vi "CC_FPGA_main.vi"() -> ()   [LabVIEW 2019]
uses:
  <vilib>/FPGAPlugInAG/sbRIO-9627/niLvFpga_Open_sbRIO-9627.vi
  <vilib>/rvi/interface/common/dynamic/niFpgaDynamicAddResources.vi
  <vilib>/Utility/error.llb/Error Cluster From Error Code.vi
  <vilib>/rvi/errors/niLvFpgaAdjustHostInterfaceError.vi
  <vilib>/FPGAPlugInAG/Dynamic/niLvFpga_Close_Dynamic.vi
  <vilib>/rvi/interface/nirviOpenFPGA/nirviOpenFPGA.xnode
  FPGA Bitfiles/ccmultiplier_FPGATarget_CCold_394fnWNrCgc.lvbitx
  CC_old.vi
  <vilib>/rvi/interface/nirviReadWriteControl/nirviReadWriteControl.xnode
  <vilib>/rvi/interface/nirviCloseFPGA/nirviCloseFPGA.xnode
  NiFpgaLv.dll
  <vilib>/rvi/interface/Simulation/niFpgaSimulationCallBeginRW.vi
panel:
  out "raw current":sgl(graph)
  in  "multiplier upper bound":sgl
  out "Loop rate current":i16
  in  "gains":T1
  out "control_ip":sgl(graph)
  out "motor direction":bool
  out "loop rate main":u32
  out "error %":sgl(knob) scale=-100.0..100.0
  out "Current control":dynamicdata(graph)
  in  "stop":bool
  in  "amplitude":sgl
  in  "Fre":sgl
  out "multiplier":sgl
  in  "weighting term motor":sgl
  in  "zero Value motor":sgl
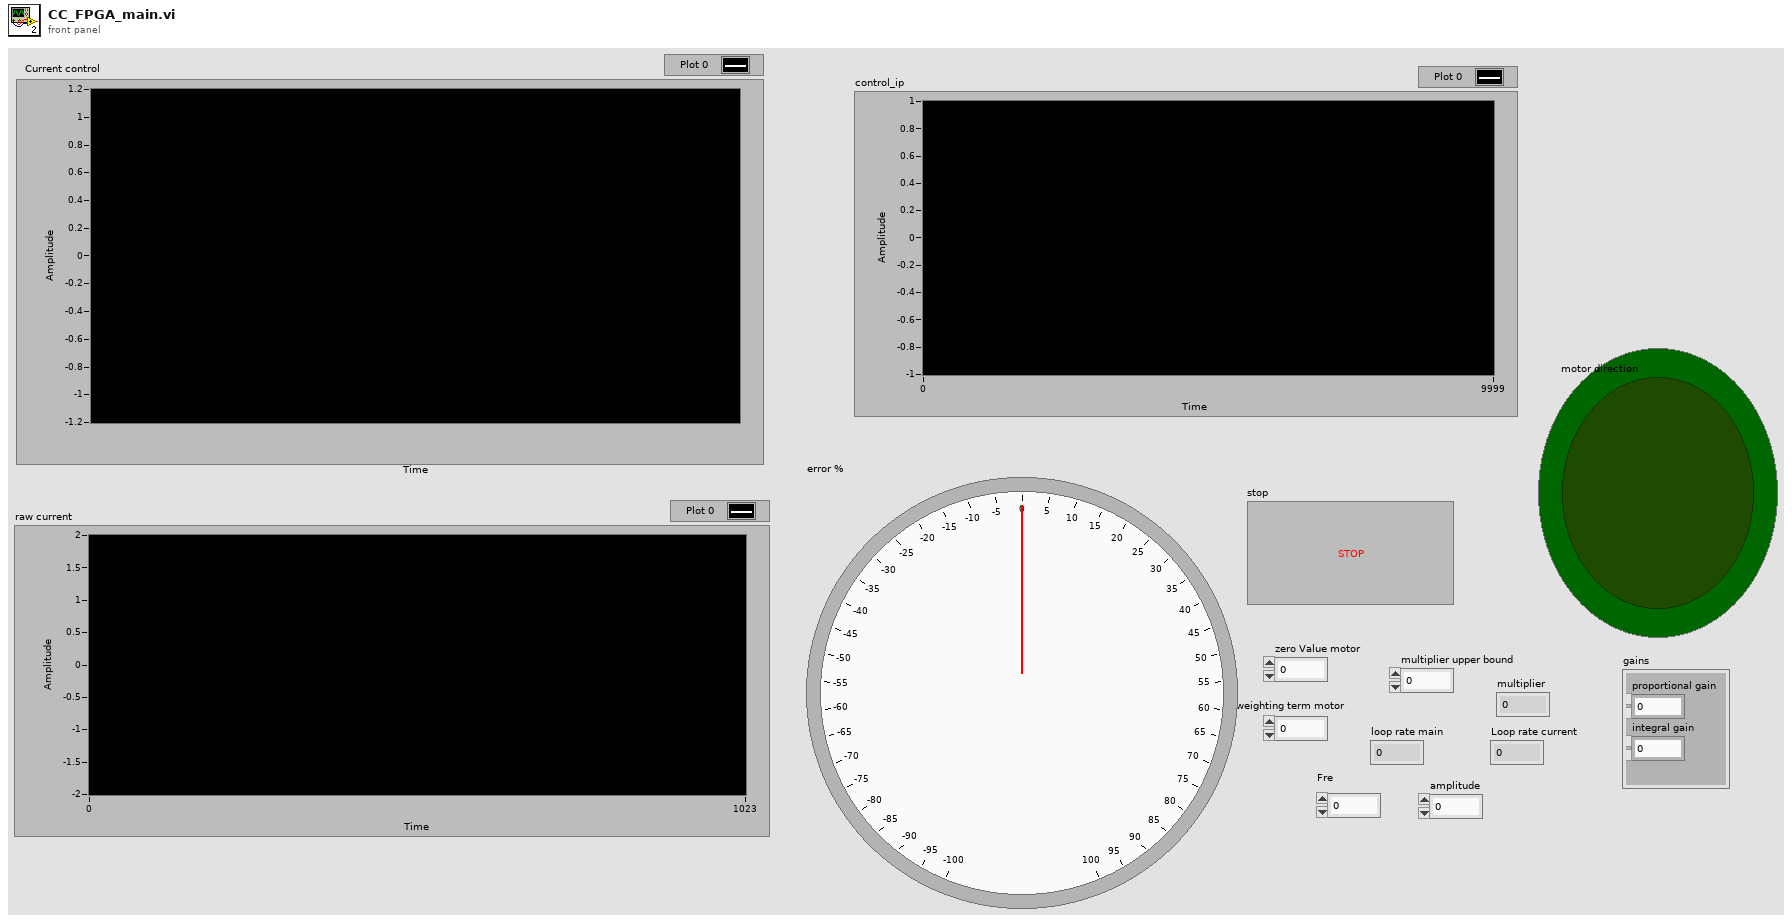
[diagram p1: front panel]
types:
  T1 = cluster{"proportional gain":sgl, "integral gain":sgl}
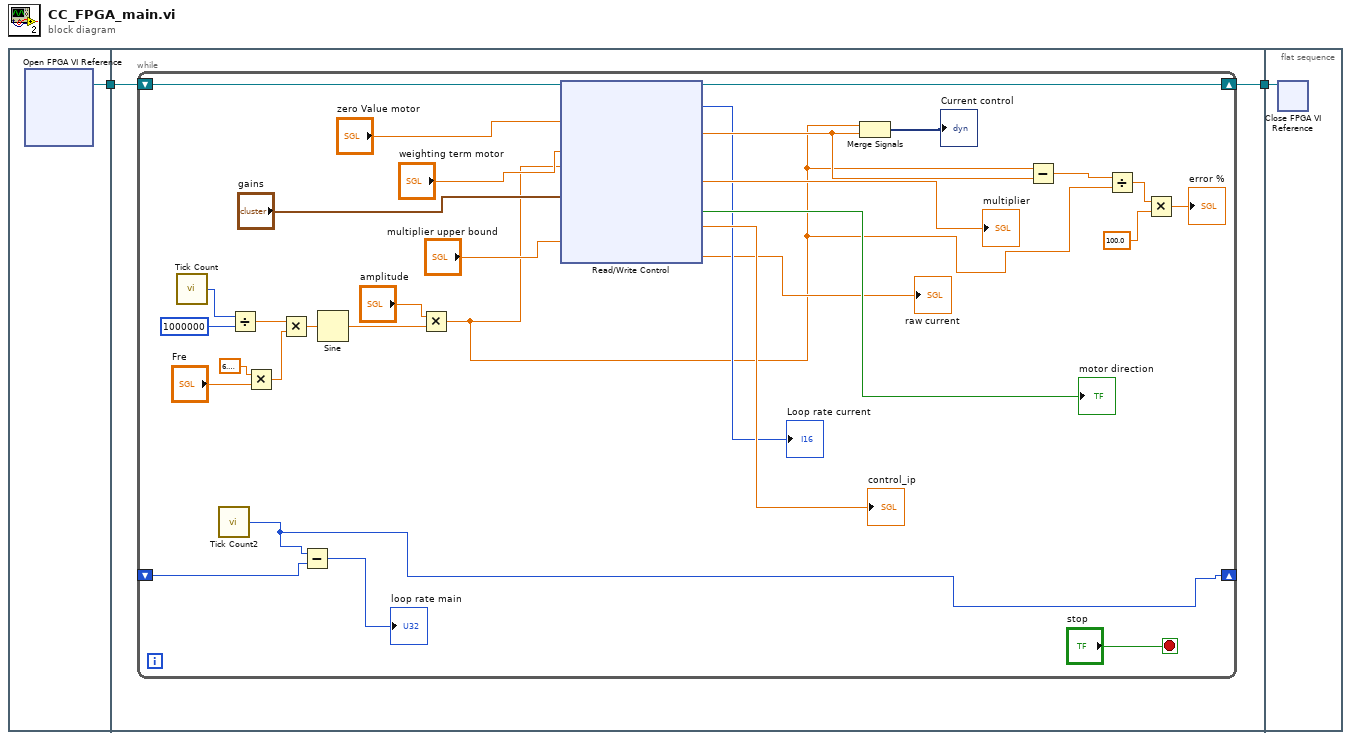
[diagram p0: block diagram]
diagram:
  n1 = flat-sequence {
    tunnel: [w3] -> w2
    tunnel: w2 -> [w5]
    tunnel: [w4] -> w1
    tunnel: w1 -> [w37]
    frame #0 {
      n2 = xnode "Open FPGA VI Reference"() -> ("FPGA VI Reference Out"=w3:refnum<k20>)  [unwired: 2 in, 1 out]
    }
    frame #1 {
      n3 = while {
        shift-right: [w35] -> w4
        shift-left: w5 -> [w36]
        shift-right: [w21] -> _
        shift-left: _ -> [w20]
        stop <- "stop" stop-if-true
        n4 = call "Tick Count"() -> ("Tick Count(uSec)"=w33:u32)
        n5 = call "Tick Count2"() -> ("Tick Count(uSec)"=w21:u32)
        n6 = Divide(x=w33, y=u32 1000000) -> (x/y=w7:dbl)
        n7 = Multiply(x=sgl 6.2831855, y="Fre") -> (x*y=w9:sgl)
        n8 = Multiply(x=w7, y=w9) -> (x*y=w31:dbl)
        n9 = Subtract(x=w21, y=w20) -> (x-y=→"loop rate main":u32)
        n10 = Sine(x=w31) -> (sin(x)=w29:dbl)
        n11 = Multiply(x="amplitude", y=w29) -> (x*y=w6:dbl)
        n12 = xnode "Read/Write Control"("FPGA VI Reference In"=w36, "zero Value M2"="zero Value motor", "weighting term(M2)"="weighting term motor", "reference"=w6, "gains"="gains", "multiplier upper bound"="multiplier upper bound") -> ("FPGA VI Reference Out"=w35:refnum<k20>, "Loop rate current"=→"Loop rate current":i16, "Filterd Current(M2)"=w17:sgl, "multiplier"=→"multiplier":sgl, "motor direction"=→"motor direction":bool, "control_ip"=→"control_ip":sgl, "raw current"=→"raw current":sgl)  [unwired: 1 in, 1 out]
        n13 = Merge Signals(w6, w17) -> (→"Current control":dynamicdata)
        n14 = Subtract(x=w6, y=w17) -> (x-y=w25:dbl)
        n15 = Divide(x=w25, y=w6) -> (x/y=w24:dbl)
        n16 = Multiply(x=w24, y=sgl 100.0) -> (x*y=→"error %":dbl)
      }
    }
    frame #2 {
      n17 = xnode "Close FPGA VI Reference"("FPGA VI Reference In"=w37) -> ()  [unwired: 1 in, 1 out]
    }
  }
